vi "ActionVIOnDelete_Good.vi"(6 "All deleted Refs":T1[](array[typedef]) format="%.0x", 8 "error in (no error)":errorcluster, 11 "Item Ref in":T1 format="%.0x") -> (0 "error out":errorcluster, 3 "Item Ref out":T1 format="%.0x")   [LabVIEW 2017]
uses:
  <vilib>/NI Veristand/Custom Device API/Custom Device Item Ref.ctl
  <vilib>/NI VeriStand/Custom Device API/Custom Device API.lvlib
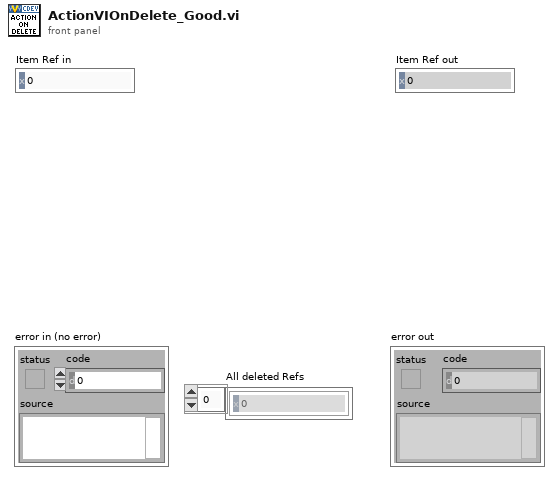
[diagram p1: front panel]
types:
  T1 = typedef "Custom Device API.lvlib/Custom Device Item Ref.ctl" = u64
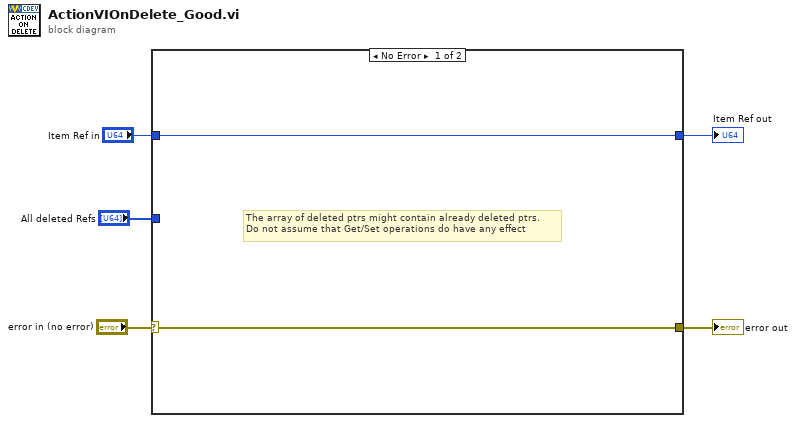
[diagram p0: block diagram]
diagram:
  n1 = case shown="No Error" "error in (no error)" {
    selector: "error in (no error)" -> [w7 w9]
    tunnel: [w7 w9] -> w4
    tunnel: "Item Ref in" -> [w6 w8]
    tunnel: [w6 w8] -> w2
    tunnel: "All deleted Refs" -> [_ _]
    frame No Error {
      # "The array of deleted ptrs might contain already deleted ptrs.\nDo not assume that Get/Set operations do have any effect"
    }
    frame Error {
    }
  }
  "error out" <- w4
  "Item Ref out" <- w2
